vi "Camera_Hamamatsu.vi"() -> ()   [LabVIEW 2014]
doc: "Allows the user to focus the camera on the sample"
uses:
  <vilib>/vision/Image Controls.llb/IMAQ Image.ctl
  <vilib>/userdefined/High Color/IMAQdx.ctl
  Widefield_globals.vi
  <vilib>/vision/NI_Vision_Development_Module.lvlib
  <vilib>/vision/driver/NI_Vision_Acquisition_Software.lvlib
  <resource>/objmgr/imaqdx.rc
panel:
  out "Binning":u16(ring) items=["1X1", "2X2", "4X4", "8X8"]
  in  "exposure time (s)":dbl
  in  "update exposure?":bool
  out "Image Buffer":T1
  out "Waveform Graph":u32[](graph)
  in  "Snap":bool
  in  "Exit Focus Loop":bool
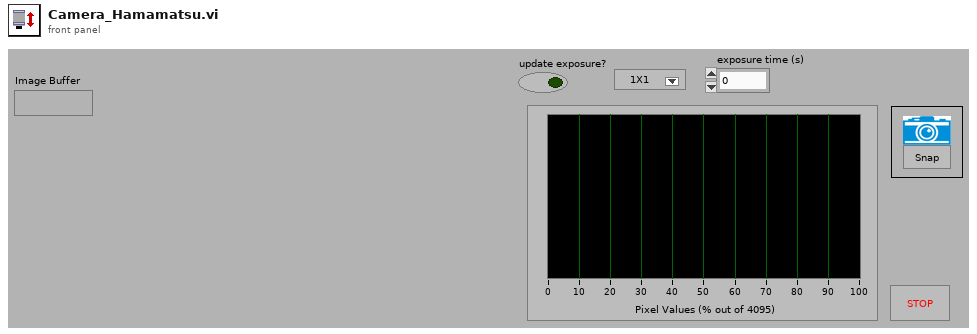
[diagram p1: front panel]
types:
  T1 = typedef "IMAQ Image.ctl" = refnum<image>
  T2 = typedef "IMAQdx.ctl" = refnum<k21>
  T3 = cluster{"histogram":u32[], "Minimal Value":sgl, "Maximal Value":sgl, "Starting Value":sgl, "Interval Width":sgl, "Mean Value":sgl, "Standard  Variation":sgl, "Area (pixels)":i32}
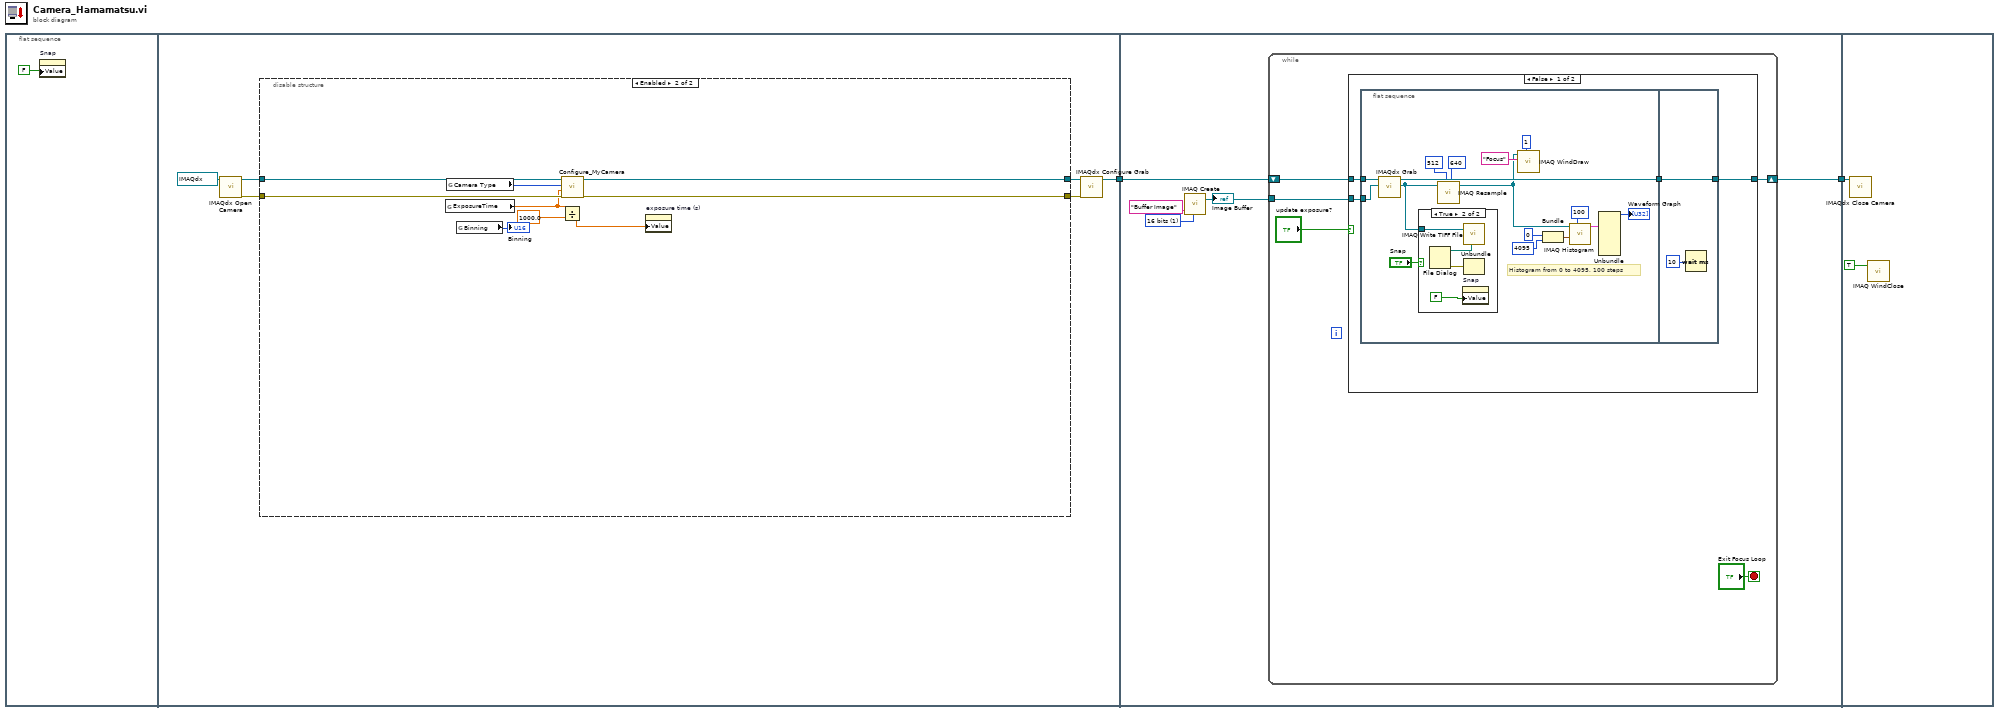
[diagram p0: block diagram]
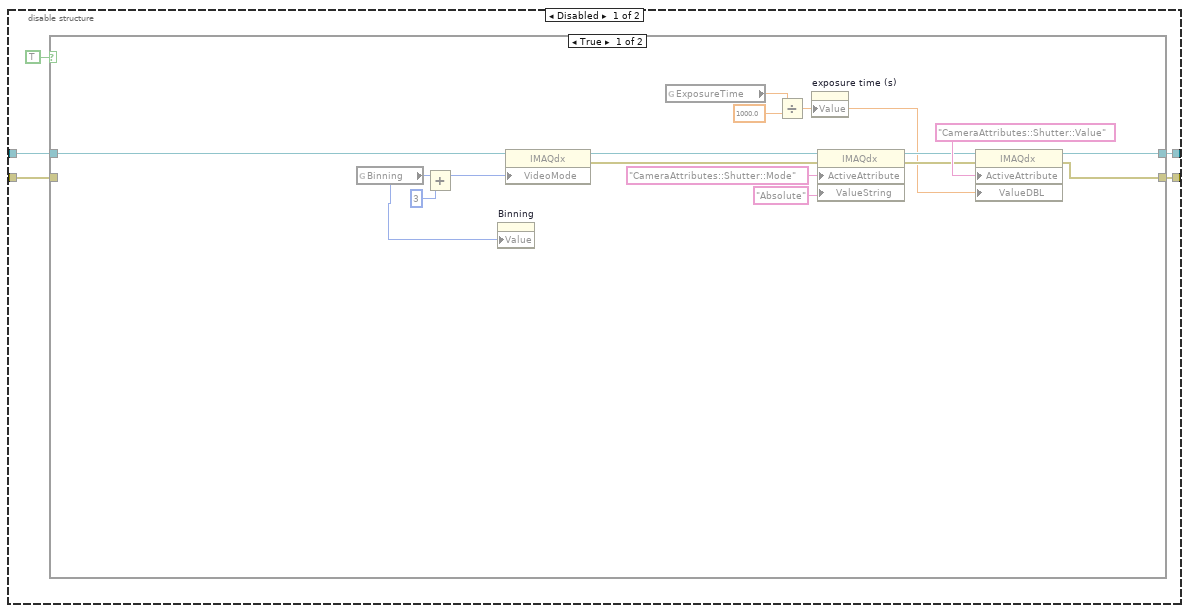
[diagram p2: hidden frame]
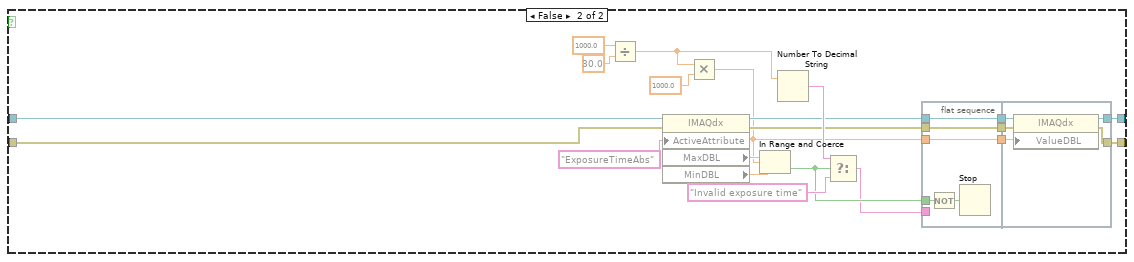
[diagram p3: hidden frame]
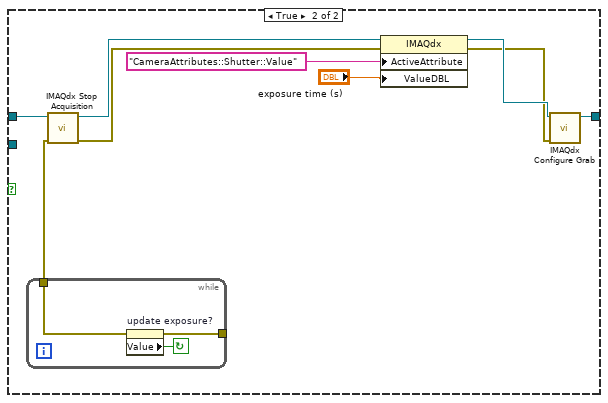
[diagram p5: hidden frame]
diagram:
  n1 = flat-sequence {
    tunnel: [w4] -> w2
    tunnel: w2 -> [w72]
    tunnel: [w71] -> w1
    tunnel: w1 -> [w118]
    frame #0 {
      n2 = property on="Snap" class="Bool (strict)"("Value"=FALSE ("Snap!")) -> ()  [unwired: 2 in, 2 out]
    }
    frame #1 {
      n3 = call <vilib>:"IMAQdx Open Camera.vi"("Session In"=T2 "cam0") -> ("error out"=w7:errorcluster, "Session Out"=w8:T2)  [unwired: 2 in, 7 out]
      n4 = disable-structure shown="Enabled" {
        disable-tunnel: [w14 w66] -> w9
        disable-tunnel: w8 -> [w13 w70]
        disable-tunnel: w7 -> [w12 w69]
        disable-tunnel: [w11 w67] -> w5
        frame Disabled {
          n5 = case shown="True" TRUE {
            tunnel: [w29 w36] -> w14
            tunnel: w13 -> [w20 w51]
            tunnel: w12 -> [_ w49]
            tunnel: [w30 w37] -> w11
            frame True {
              n6 = global read "Widefield_globals.vi" "Binning"() -> (w15:u16)
              n7 = Add(x=w15, y=u16 3) -> (x+y=w17:u16)
              n8 = property on="Binning" class="Ring (strict)"("Value"=w15) -> ()  [unwired: 2 in, 2 out]
              n9 = property class="IMAQdx"(reference=w20, "VideoMode"=w17) -> (reference out=w19:T2, error out=w18:errorcluster)  [unwired: 1 in]
              n10 = global read "Widefield_globals.vi" "ExposureTime"() -> (w26:dbl)
              n11 = Divide(x=w26, y=1000.0) -> (x/y=w21:dbl)
              n12 = property on="exposure time (s)" class="DigNum (strict)"("Value"=w21) -> ()  [unwired: 2 in, 2 out]
              n13 = property class="IMAQdx"(reference=w19, error in=w18, "ActiveAttribute"="CameraAttributes::Shutter::Mode", "ValueString"="Absolute") -> (reference out=w23:T2, error out=w24:errorcluster)
              n14 = property class="IMAQdx"(reference=w23, error in=w24, "ActiveAttribute"="CameraAttributes::Shutter::Value", "ValueDBL"=w21) -> (reference out=w30:T2, error out=w29:errorcluster)
            }
            frame False {
              n15 = Divide(x=1000.0 ("y"), y=30.0) -> (x/y=w32:dbl)
              n16 = property class="IMAQdx"(reference=w51, error in=w49, "ActiveAttribute"="ExposureTimeAbs" ("Camera Attribute")) -> (reference out=w43:T2, error out=w42:errorcluster, "MaxDBL"=w48:dbl, "MinDBL"=w35:dbl)
              n17 = Multiply(x=w32, y=1000.0) -> (x*y=w38:dbl)
              n18 = In Range and Coerce(upper limit=w48, x=w38, lower limit=w35) -> (In Range?=w44:bool)  [unwired: 1 out]
              n19 = Number To Decimal String(number=w32) -> (decimal integer string=w45:string)  [unwired: 1 out]
              n20 = Select(t=w45, s=w44, f="Invalid exposure time") -> (s? t:f=w31:string)
              n21 = flat-sequence {
                tunnel: w31 -> [_]
                tunnel: w44 -> [w55]
                tunnel: w43 -> [w53]
                tunnel: w42 -> [w54]
                tunnel: [w54] -> w41
                tunnel: [w53] -> w40
                tunnel: [w52] -> w39
                tunnel: w38 -> [w52]
                tunnel: w41 -> [w60]
                tunnel: w40 -> [w61]
                tunnel: w39 -> [w59]
                tunnel: [w58] -> w37
                tunnel: [w57] -> w36
                frame #0 {
                  n22 = Not(x=w55) -> (.not. x?=w56:bool)
                  n23 = Stop(stop? (T)=w56) -> ()
                }
                frame #1 {
                  n24 = property class="IMAQdx"(reference=w61, error in=w60, "ValueDBL"=w59) -> (reference out=w58:T2, error out=w57:errorcluster)
                }
              }
            }
          }
        }
        frame Enabled {
          n25 = global read "Widefield_globals.vi" "ExposureTime"() -> (w65:dbl)
          n26 = global read "Widefield_globals.vi" "Camera Type"() -> (w62:u16)
          n27 = global read "Widefield_globals.vi" "Binning"() -> (→"Binning":u16)
          n28 = call "Configure_MyCamera.vi"("Camera Error In"=w69, "ExposureTime (ms)"=w65, "Camera Type"=w62, "Camera Session In"=w70) -> ("Camera Error Out"=w66:errorcluster, "Camera Session Out"=w67:T2)  [unwired: 2 in]
          n29 = Divide(x=w65, y=1000.0) -> (x/y=w64:dbl)
          n30 = property on="exposure time (s)" class="DigNum (strict)"("Value"=w64) -> ()  [unwired: 2 in, 2 out]
        }
      }
      n31 = call <vilib>:"IMAQdx Configure Grab.vi"("error in"=w9, "Session In"=w5) -> ("Session Out"=w4:T2)  [unwired: 9 out]
    }
    frame #2 {
      w74 = u32 1 items=["8 bits", "16 bits", "Float", "Complex", "RGB", "HSL"] ("Image Type")
      n32 = call "IMAQ Create"("Image Name"="Buffer Image", "Image Type"=w74) -> ("New Image"=w73:T1)  [unwired: 2 in, 2 out]
      "Image Buffer" <- w73
      n33 = while {
        tunnel: w73 -> [w79]
        shift-right: [w76] -> w71
        shift-left: w72 -> [w78]
        stop <- "Exit Focus Loop" stop-if-true
        n34 = case shown="False" "update exposure?" {
          tunnel: w79 -> [w83 _]
          tunnel: [w82 w115] -> w76
          tunnel: w78 -> [w81 w114]
          frame False {
            n35 = flat-sequence {
              tunnel: w83 -> [w91]
              tunnel: [w90] -> w84
              tunnel: w81 -> [w89]
              tunnel: [w105] -> w82
              tunnel: w84 -> [w105]
              frame #0 {
                # "Histogram from 0 to 4095, 100 steps"
                n36 = call <vilib>:"IMAQdx Grab.vi"("Image In"=w91, "Session In"=w89) -> ("Image Out"=w86:T1, "Session Out"=w90:T2)  [unwired: 2 in, 6 out]
                n37 = case shown="True" "Snap" {
                  tunnel: w86 -> [_ w103]
                  frame False {
                  }
                  frame True {
                    n38 = File Dialog() -> (0:w102:errorcluster, 3:w104:path)  [unwired: 1 in, 8 out]
                    n39 = property on="Snap" class="Bool (strict)"("Value"=FALSE ("Snap!")) -> ()  [unwired: 2 in, 2 out]
                    n40 = call "IMAQ Write TIFF File"("File Path"=w104, "Image"=w103) -> ()  [unwired: 3 in, 4 out]
                    n41 = Unbundle(w102) -> ()  [unwired: 3 out]
                  }
                }
                n42 = call "IMAQ Resample"("X Resolution"=640, "Y Resolution"=512, "Image Src"=w86) -> ("Image Dst Out"=w85:T1)  [unwired: 4 in, 4 out]
                n43 = call "IMAQ WindDraw"("Window Number (0...15)"=1, "Title"="Focus", "Image"=w85) -> ()  [unwired: 3 in, 6 out]
                n44 = Bundle(0, 4095) -> (w92:cluster{i32, i32})  [unwired: 1 out]
                n45 = call "IMAQ Histogram"("Number of Classes"=100, "Interval Range"=w92, "Image"=w85) -> ("Histogram Report"=w97:T3)  [unwired: 2 in, 6 out]
                n46 = Unbundle(w97) -> ("histogram"=→"Waveform Graph":u32[])  [unwired: 7 out]
              }
              frame #1 {
                n47 = Wait (ms)(milliseconds to wait=u32 10) -> ()  [unwired: 1 out]
              }
            }
          }
          frame True {
            n48 = while {
              tunnel: [w116] -> _
              tunnel: [w116] -> w111
              stop <- w117 continue-if-true
              n49 = property on="update exposure?" class="Bool (strict)"() -> (error out=w116:errorcluster, "Value"=w117:bool)  [unwired: 2 in, 1 out]
            }
            n50 = call <vilib>:"IMAQdx Stop Acquisition.vi"("error in"=w111, "Session In"=w114) -> ("error out"=w110:errorcluster, "Session Out"=w113:T2)  [unwired: 8 in]
            n51 = property class="IMAQdx"(reference=w113, error in=w110, "ActiveAttribute"="CameraAttributes::Shutter::Value", "ValueDBL"="exposure time (s)") -> (reference out=w112:T2, error out=w109:errorcluster)
            n52 = call <vilib>:"IMAQdx Configure Grab.vi"("error in"=w109, "Session In"=w112) -> ("Session Out"=w115:T2)  [unwired: 9 out]
          }
        }
      }
    }
    frame #3 {
      n53 = call <vilib>:"IMAQdx Close Camera.vi"("Session In"=w118) -> ()  [unwired: 1 in, 10 out]
      n54 = call "IMAQ WindClose"("Close All Windows (False)"=TRUE) -> ()  [unwired: 2 in, 4 out]
    }
  }
